vi "Thermo_stop.vi"(8 "error in (no error)":errorcluster, 11 "VISA resource name":refnum<visa-resource-name>) -> (0 "error out":errorcluster, 3 "VISA resource name out":refnum<visa-resource-name>)   [LabVIEW 2015]
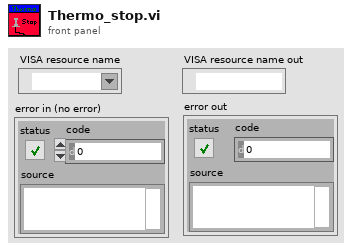
[diagram p1: front panel]
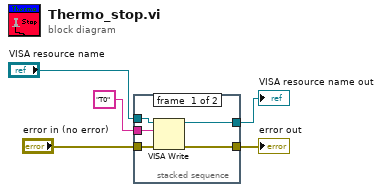
[diagram p0: block diagram]
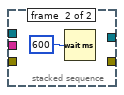
[diagram p2: hidden frame]
diagram:
  n1 = stacked-sequence {
    tunnel: "VISA resource name" -> [w10 _]
    tunnel: "T0" -> [w9 _]
    tunnel: "error in (no error)" -> [w8 _]
    tunnel: [w7 _] -> w2
    tunnel: [w6 _] -> w1
    frame #0 {
      n2 = VISA Write(VISA resource name=w10, write buffer=w9, error in (no error)=w8) -> (VISA resource name out=w6:refnum<visa-resource-name>, error out=w7:errorcluster)  [unwired: 1 out]
    }
    frame #1 {
      n3 = Wait (ms)(milliseconds to wait=600) -> ()  [unwired: 1 out]
    }
  }
  "error out" <- w2
  "VISA resource name out" <- w1
